vi "Register Events and Run.vi"(8 "error in (no error)":errorcluster, 11 "Panel in":refnum<class "Panel.lvclass">) -> (0 "error out":errorcluster, 2 "Panel Event Reg":refnum<event-registration>, 3 "Panel out":refnum<class "Panel.lvclass">)   [LabVIEW 2014, in "OOPanel.lvlib" / "Panel.lvclass"]
uses:
  Panel.lvclass
  Visibility State.ctl
  Visbility Event Data.ctl
  Close Reason.ctl
  Panel Events.ctl
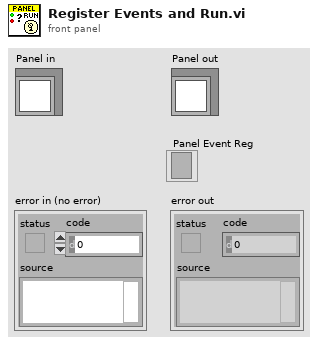
[diagram p1: front panel]
types:
  T1 = typedef "OOPanel.lvlib/Panel.lvclass/Ref Data.ctl" = cluster{"Panel Events":T2, "Panel Ref":refnum<vi>, "SubPanel":refnum<vi>, "Close":bool, "Running":bool, "State":T3}
  T2 = typedef "OOPanel.lvlib/Panel.lvclass/Panel Events.ctl" = cluster{"Visbility":refnum<user-event>, "Close":refnum<user-event>}
  T3 = typedef "OOPanel.lvlib/Panel.lvclass/Visibility State.ctl" = enum16{"Idle", "Closed", "Hidden", "Visible", "Subpanel"}
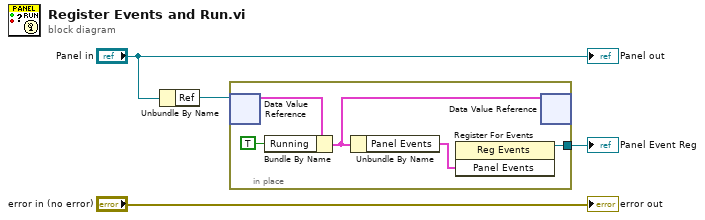
[diagram p0: block diagram]
diagram:
  n1 = Unbundle By Name("Panel in") -> ("Ref"=w3:refnum<data-value>)
  n2 = in-place {
    in-place-border: [w5] -> w1
    n3 = in-place-dvr #1(w3) -> (w9:T1)  [unwired: 1 out]
    n4 = Bundle By Name(cluster=w9, "Running"=TRUE) -> (w7:T1)
    n5 = Unbundle By Name(w7) -> ("Panel Events"=w6:T2)
    n6 = register-events(w6) -> (reference out=w5:refnum<event-registration>)  [unwired: 2 in, 1 out]
    n7 = in-place-dvr #1(w7) -> ()  [unwired: 2 out]
  }
  "Panel Event Reg" <- w1
  "error out" <- "error in (no error)"
  "Panel out" <- "Panel in"
